vi "Read Patch.vi"(8 "error in (no error)":errorcluster, 11 "Semver in":refnum<class "Semver.lvclass">) -> (0 "error out":errorcluster, 2 "Patch":i32, 3 "Semver out":refnum<class "Semver.lvclass">)   [LabVIEW 2017, in "Semver.lvlib" / "Semver.lvclass"]
uses:
  Semver.lvclass
  Semver.lvclass/Semver.ctl
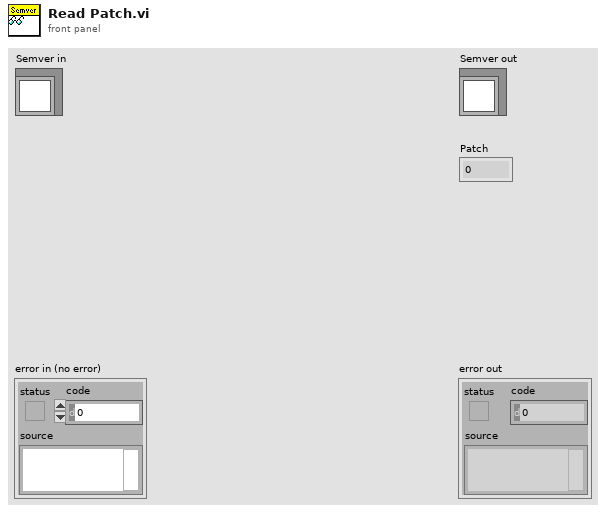
[diagram p1: front panel]
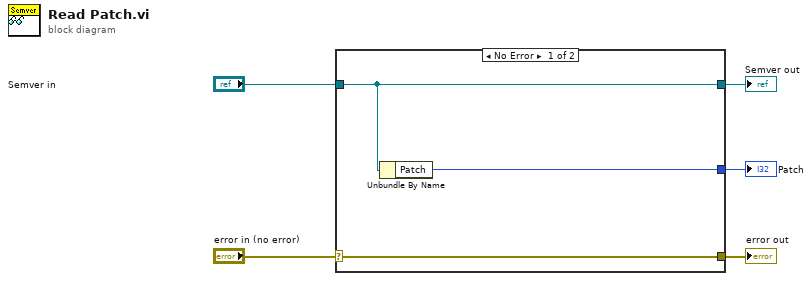
[diagram p0: block diagram]
diagram:
  n1 = case shown="No Error" "error in (no error)" {
    selector: "error in (no error)" -> [w8 w9]
    tunnel: [w8 w9] -> w4
    tunnel: [w7 w10] -> w2
    tunnel: "Semver in" -> [w7 w10]
    tunnel: [w6 _] -> w1
    frame No Error {
      n2 = Unbundle By Name(w7) -> ("Patch"=w6:i32)
    }
    frame Error {
    }
  }
  "error out" <- w4
  "Semver out" <- w2
  "Patch" <- w1
